vi "Nil.vi"() -> (1 "msgpack null":u8)   [LabVIEW 2020, in "wamplv.lvlib" / "MessagePack.lvclass"]
uses:
  MessagePack.lvclass
  MessagePack.lvclass/MessagePack.ctl
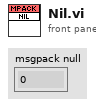
[diagram p1: front panel]
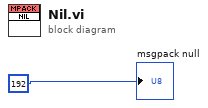
[diagram p0: block diagram]
diagram:
  "msgpack null" <- u8 192
